vi "Assert_IsFile.vi"(10 "body":string) -> (2 "File":path, 3 "is File?":bool)   [LabVIEW 2013, in "REST Client.lvlib" / "REST Client.lvclass"]
uses:
  REST Client.lvclass
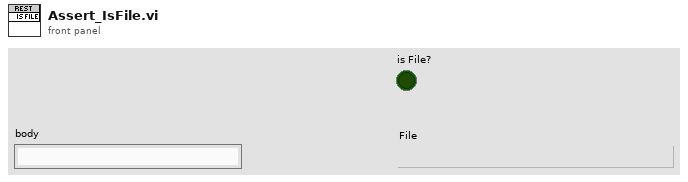
[diagram p1: front panel]
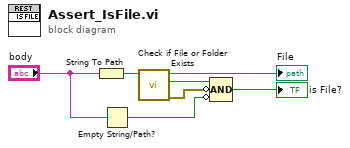
[diagram p0: block diagram]
diagram:
  n1 = String To Path(string="body") -> (path=w6:path)
  n2 = Empty String/Path?(string/path="body") -> (empty?=w3:bool)
  n3 = call <vilib>:"Check if File or Folder Exists.vi"("path"=w6) -> ("error out"=w4:errorcluster, "file or folder exists?"=w5:bool, "dup path"=→"File":path)  [unwired: 8 in]
  n4 = Compound Arithmetic op=AND(w5, invert w4, invert w3) -> (→"is File?":bool)
